vi "Eat.vi"(11 "Snake in":refnum<class "Snake.lvclass">) -> (3 "Snake out":refnum<class "Snake.lvclass">)   [LabVIEW 2020, in "Snake.lvclass"]
uses:
  Snake.lvclass
  Snake.lvclass/Snake.ctl
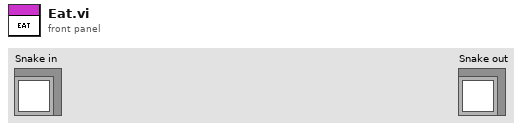
[diagram p1: front panel]
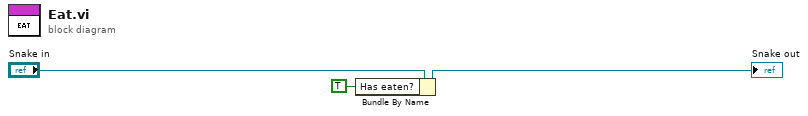
[diagram p0: block diagram]
diagram:
  n1 = Bundle By Name(cluster="Snake in", "Has eaten?"=TRUE) -> (→"Snake out":refnum<class "Snake.lvclass">)
